vi "Queue Receive.vi"(11 "jettl Queue Actor in":refnum<class "jettl Queue Actor.lvclass">) -> (2 "Msg":refnum<class "Msg.lvclass">, 3 "jettl Queue Actor out":refnum<class "jettl Queue Actor.lvclass">)   [LabVIEW 2021, in "jettl.lvlib" / "jettl Queue Actor.lvlib" / "jettl Queue Actor.lvclass"]
uses:
  jettl Queue Actor.lvclass
  Actor/Msg/Msg.lvclass
  jettl Queue Actor.lvclass/jettl Queue Actor.ctl
  jettl.lvlib
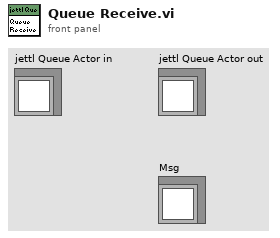
[diagram p1: front panel]
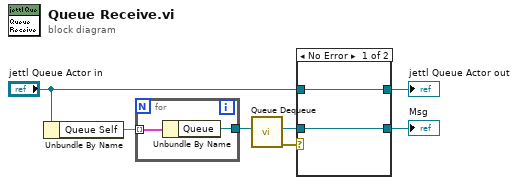
[diagram p0: block diagram]
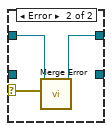
[diagram p2: hidden frame]
diagram:
  n1 = Unbundle By Name("jettl Queue Actor in") -> ("Queue Self"=w2:map{string, refnum<data-value>})
  n2 = for {
    tunnel: w2 -> [w9] mode=indexing
    tunnel: [w8] -> w1
    n3 = Unbundle By Name(w9) -> ("Queue"=w8:refnum<data-value>)
  }
  n4 = call "Queue Dequeue.vi"("Queue"=w1) -> ("error out"=w7:errorcluster, "Msg"=w6:refnum<class "Msg.lvclass">)  [unwired: 9 in]
  n5 = case shown="No Error" w7 {
    selector: w7 -> [_ w12]
    tunnel: w6 -> [w10 _]
    tunnel: "jettl Queue Actor in" -> [w11 w14]
    tunnel: [w11 w13] -> w5
    tunnel: [w10 _] -> w4
    frame No Error {
    }
    frame Error {
      n6 = call-dynamic "Merge Error.vi"("Error"=w12, "jettl Queue Actor in"=w14) -> ("jettl Queue Actor out"=w13:refnum<class "jettl Queue Actor.lvclass">)  [unwired: 9 in]
    }
  }
  "jettl Queue Actor out" <- w5
  "Msg" <- w4
